vi "Accelerometer_status_2.vi"(6 "Number":i32, 8 "Pattern frequency (Hz)":dbl=159.2, 9 "Frecuencia de muestreo (Hz)":dbl=25600.0, 10 "Acc_offset":dbl=0.004, 11 "Accelerometer":sgl[](array[numeric])=array[5000 elements]) -> (2 "Accelerometer_status":string, 3 "Accelerometer":bool)   [LabVIEW 2015]
uses:
  <vilib>/Analysis/5stat.llb/RMS (DBL).vi
  <vilib>/measure/madcrms.llb/Basic Averaged DC-RMS for 1 Chan.vi
  <vilib>/measure/NI_MAPro.lvlib
  <vilib>/Analysis/NI_AALPro.lvlib
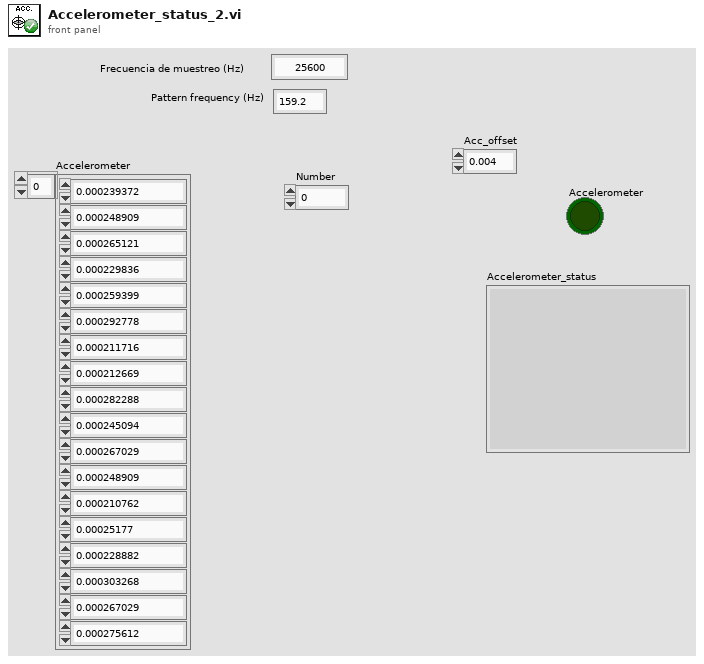
[diagram p1: front panel]
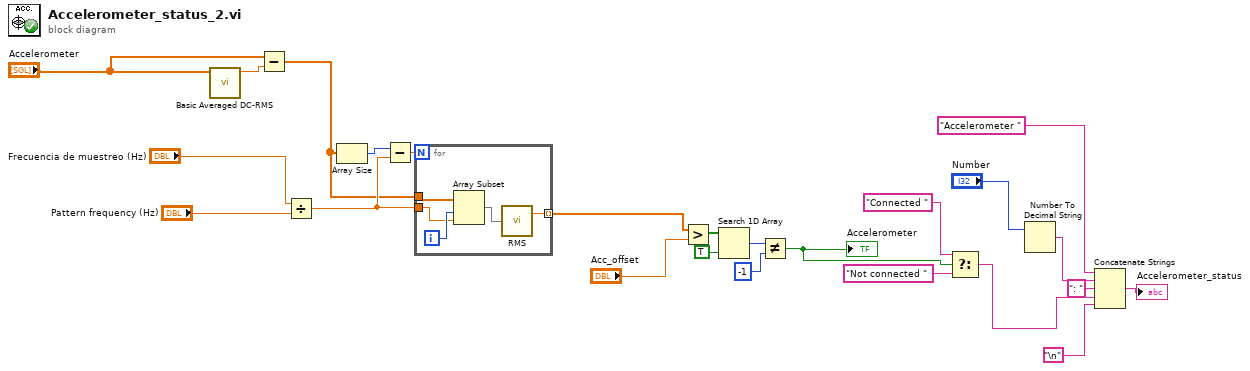
[diagram p0: block diagram]
diagram:
  n1 = call-poly <vilib>:"Basic Averaged DC-RMS.vi"("signal in"="Accelerometer") -> ("DC value"=w11:dbl)  [unwired: 7 in, 3 out]
  n2 = Subtract(x="Accelerometer", y=w11) -> (x-y=w12:dbl[])
  n3 = Divide(x="Frecuencia de muestreo (Hz)", y="Pattern frequency (Hz)") -> (x/y=w13:dbl)
  n4 = Array Size(array=w12) -> (size(s)=w14:i32)
  n5 = Subtract(x=w14, y=w13) -> (x-y=w15:dbl)
  n6 = for {
    N: w15 -> [_]
    tunnel: w13 -> [w26]
    tunnel: [w29] -> w5 mode=indexing
    tunnel: w12 -> [w28]
    i -> [w27]
    n7 = Array Subset(array=w28, index=w27, length=w26) -> (w25:dbl[])
    n8 = call-poly <vilib>:"RMS.vi"("X"=w25) -> ("rms value"=w29:dbl)  [unwired: 1 out]
  }
  n9 = Greater?(x=w5, y="Acc_offset") -> (0:w9:bool[])
  n10 = Search 1D Array(1D array=w9, element=TRUE) -> (index of element=w7:i32)  [unwired: 1 in]
  n11 = Not Equal?(x=w7, y=-1) -> (x != y?=w3:bool)
  "Accelerometer" <- w3
  n12 = Select(t="Connected " ("string"), s=w3, f="Not connected " ("string")) -> (s? t:f=w22:string)
  n13 = Number To Decimal String(number="Number") -> (decimal integer string=w17:string)  [unwired: 1 in]
  n14 = Concatenate Strings("Accelerometer " ("string"), w17, ": " ("string"), w22, "\n") -> (→"Accelerometer_status":string)
